vi "DSF.Engine.Sequencer.Set Plugin Timings.vi"(8 "error in (no error)":errorcluster, 10 "Plugin Timings":refnum<class "DSF.Engine.Timing.lvclass">[](array[class]), 11 "Sequencer in":refnum<class "DSF.Engine.Sequencer.lvclass">) -> (0 "error out":errorcluster, 3 "Sequencer out":refnum<class "DSF.Engine.Sequencer.lvclass">)   [LabVIEW 2016, in "DSF.Engine.lvlib" / "DSF.Engine.Sequencer.lvclass"]
uses:
  DSF.Engine.Sequencer.lvclass
  Timing/DSF.Engine.Timing.lvclass
  DSF.Engine.Sequencer.lvclass/DSF.Engine.Sequencer.ctl
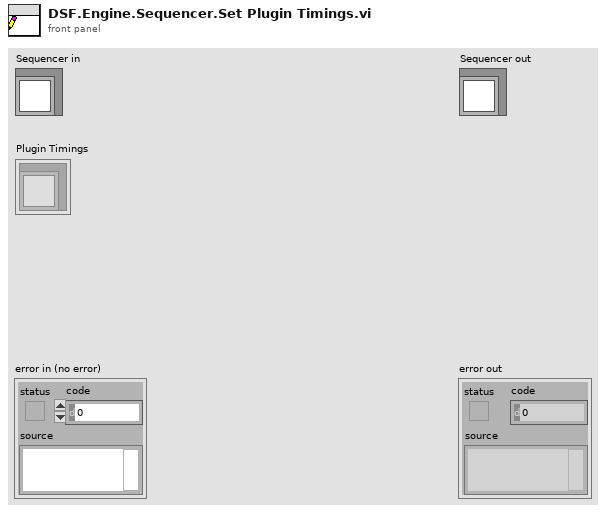
[diagram p1: front panel]
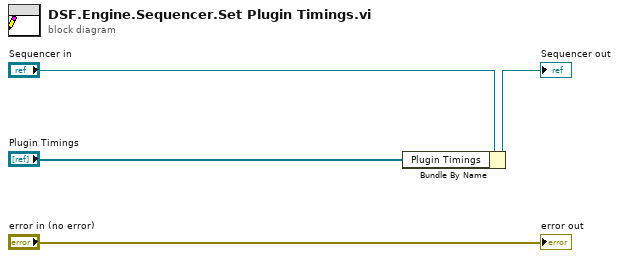
[diagram p0: block diagram]
diagram:
  n1 = Bundle By Name(cluster="Sequencer in", "Plugin Timings"="Plugin Timings") -> (→"Sequencer out":refnum<class "DSF.Engine.Sequencer.lvclass">)
  "error out" <- "error in (no error)"
